vi "MasterSlaveDAQ-SplitSlave.vi"() -> ()   [LabVIEW 2014]
uses:
  subVIs/SlaveState.ctl
  subVIs/SlaveStateData.ctl
  <vilib>/Utility/error.llb/DialogType.ctl
  <vilib>/DAQmx/read.llb/DAQmx Read (Analog Wfm 1Chan NSamp).vi
  <resource>/objmgr/daqmx.rc
panel:
  out "Waveform Chart":waveform(dbl)(graph)
  in  "Acquire Data":bool
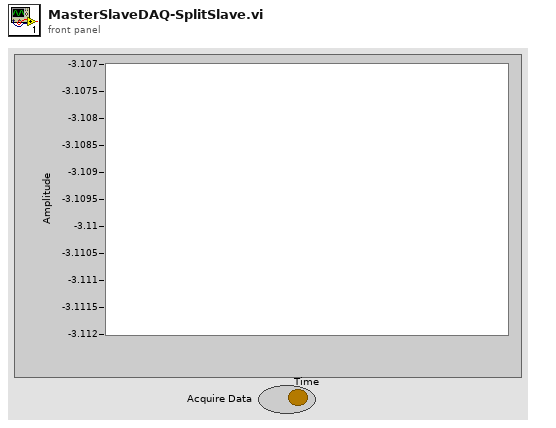
[diagram p1: front panel]
types:
  T1 = typedef "SlaveStateData.ctl" = cluster{"New State":T2, "DAQ Ref":refnum<k21>, "File Ref":refnum<file>}
  T2 = typedef "SlaveState.ctl" = enum16{"Init", "Idle", "CheckError", "Finalize", "StartDAQ", "AcquireAndLog", "StopDAQ", "UpdateFile"}
  T3 = typedef "DialogType.ctl" = u16
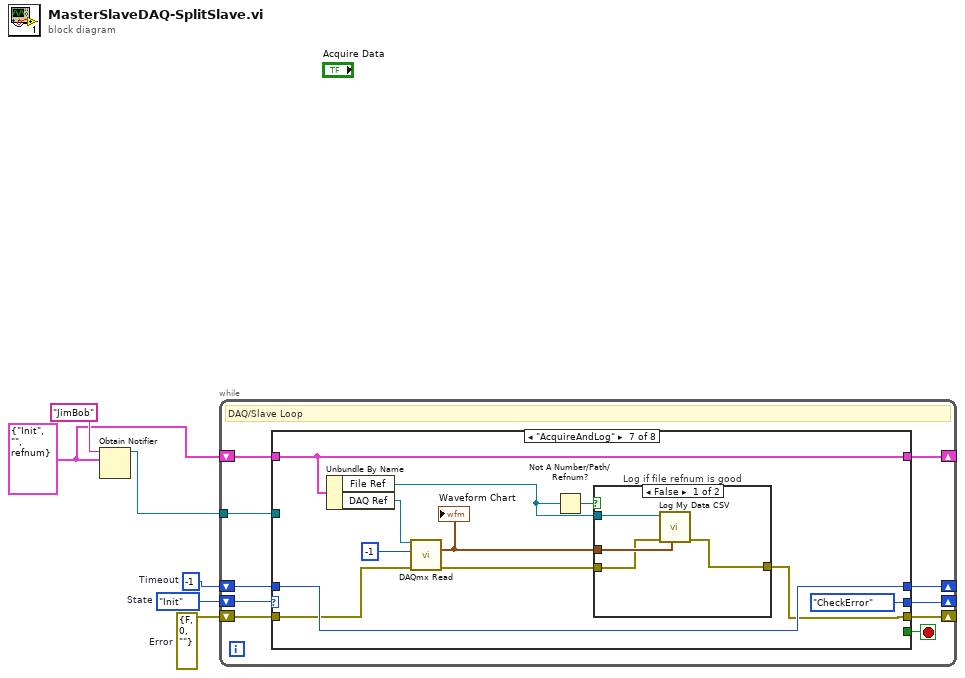
[diagram p0: block diagram]
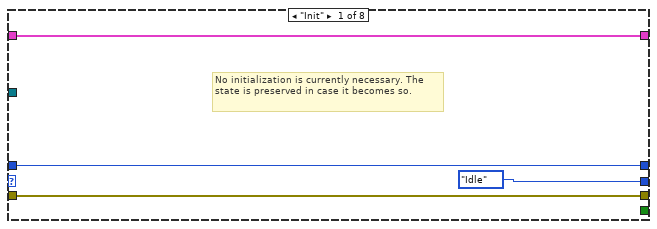
[diagram p2: hidden frame]
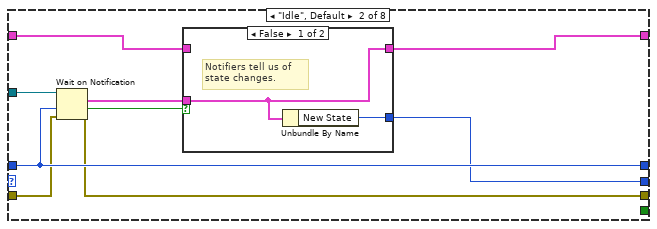
[diagram p3: hidden frame]
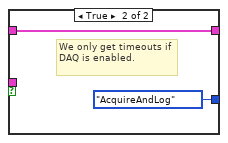
[diagram p4: hidden frame]
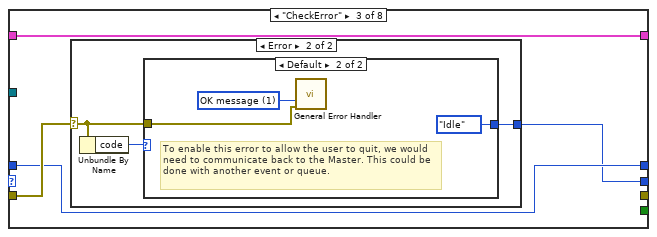
[diagram p5: hidden frame]
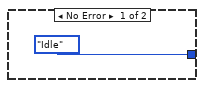
[diagram p6: hidden frame]
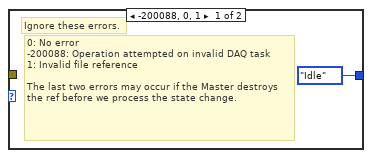
[diagram p7: hidden frame]
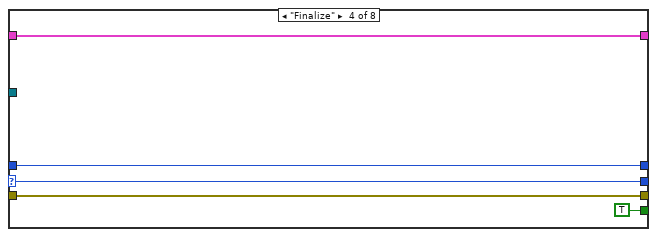
[diagram p8: hidden frame]
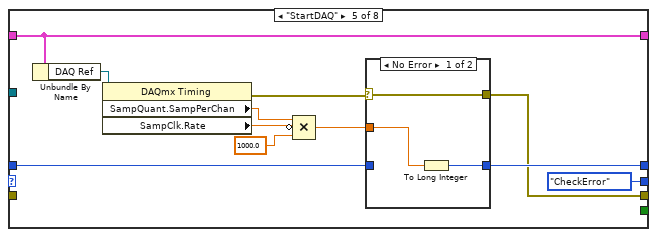
[diagram p9: hidden frame]
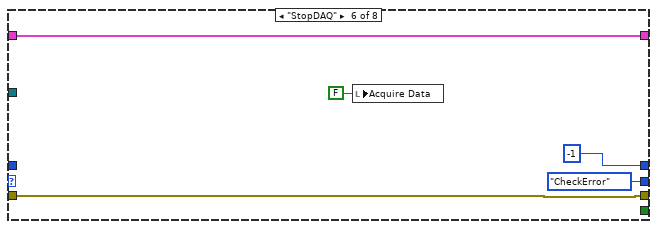
[diagram p11: hidden frame]
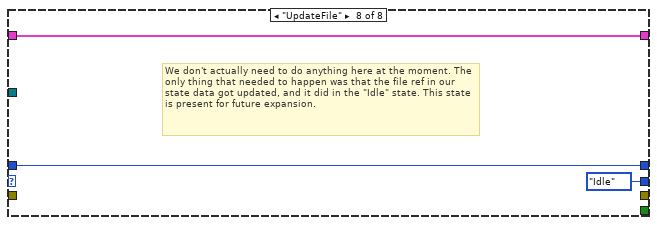
[diagram p13: hidden frame]
diagram:
  w1 = T1 {"New State"=enum."Init", "DAQ Ref"="", "File Ref"=refnum}
  w4 = errorcluster {"status"=FALSE, "code"=0, "source"=""}  # Error
  w5 = -1  # Timeout
  w6 = SlaveState."Init"  # State
  n1 = Obtain Notifier(name (unnamed)="JimBob", notification data type=w1) -> (notifier out=w2:refnum<notifier>)  [unwired: 2 in, 2 out]
  n2 = while {
    tunnel: w2 -> [w15]
    shift-right: [w14] -> _
    shift-left: w6 -> [w16]
    shift-right: [w10] -> _
    shift-left: w1 -> [w13]
    shift-right: [w11] -> _
    shift-left: w5 -> [w12]
    shift-right: [w8] -> _
    shift-left: w4 -> [w9]
    stop <- w7 stop-if-true
    # "DAQ/Slave Loop"
    n3 = case shown="\"AcquireAndLog\"" w16 {
      selector: w16 -> [_ _ _ w47 _ _ _ _]
      tunnel: w15 -> [_ w29 _ _ _ _ _ _]
      tunnel: [SlaveState."Idle" ("New State") w22 w34 w47 SlaveState."CheckError" ("State") SlaveState."CheckError" ("State") SlaveState."CheckError" ("State") SlaveState."Idle" ("State")] -> w14
      tunnel: w13 -> [w18 w24 w37 w49 w58 w71 w76 w90]
      tunnel: w12 -> [w19 w28 w35 w48 w60 _ w77 w89]
      tunnel: [w19 w28 w35 w48 w61 -1 w77 w89] -> w11
      tunnel: [w18 w21 w37 w49 w58 w71 w76 w90] -> w10
      tunnel: w9 -> [w17 w26 w36 w46 _ w67 w74 _]
      tunnel: [w17 w27 _ w46 w59 w67 w73 _] -> w8
      tunnel: [_ _ _ TRUE _ _ _ _] -> w7
      frame "Init" {
        # "No initialization is currently necessary. The state is preserved in case it becomes so."
      }
      frame "Idle", Default {
        n4 = Wait on Notification(notifier=w29, timeout in ms (-1)=w28, error in (no error)=w26) -> (notification=w23:T1, timed out?=w25:bool, error out=w27:errorcluster)  [unwired: 1 in, 1 out]
        n5 = case shown="False" w25 {
          tunnel: w24 -> [_ w33]
          tunnel: w23 -> [w30 _]
          tunnel: [w31 SlaveState."AcquireAndLog" ("New State")] -> w22
          tunnel: [w30 w33] -> w21
          frame False {
            # "Notifiers tell us of state changes."
            n6 = Unbundle By Name(w30) -> ("New State"=w31:T2)
          }
          frame True {
            # "We only get timeouts if DAQ is enabled."
          }
        }
      }
      frame "CheckError" {
        n7 = case shown="Error" w36 {
          selector: w36 -> [_ w40]
          tunnel: [SlaveState."Idle" ("State") w41] -> w34
          frame No Error {
          }
          frame Error {
            n8 = Unbundle By Name(w40) -> ("code"=w39:i32)
            n9 = case shown="Default" w39 {
              tunnel: [SlaveState."Idle" ("State") SlaveState."Idle" ("State")] -> w41
              tunnel: w40 -> [_ w44]
              frame -200088, 0, 1 {
                # "0: No error\n-200088: Operation attempted on invalid DAQ task\n1: Invalid file reference\n\nThe last two errors may occur if the Master destroys the ref before we process the state change."
                # "Ignore these errors."
              }
              frame Default {
                w45 = T3 1 items=["no dialog", "OK message", "continue or stop message", "OK message + warnings", "continue/stop + warnings"] ("type of dialog (OK msg:1)")
                # "To enable this error to allow the user to quit, we would need to communicate back to the Master. This could be done with another event or queue."
                n10 = call <vilib>:"General Error Handler.vi"("type of dialog (OK msg:1)"=w45, "error in (no error)"=w44) -> ()  [unwired: 9 in, 5 out]
              }
            }
          }
        }
      }
      frame "Finalize" {
      }
      frame "StartDAQ" {
        n11 = Unbundle By Name(w58) -> ("DAQ Ref"=w57:refnum<k21>)
        n12 = property class="DAQmx Timing"(reference=w57) -> (error out=w55:errorcluster, "SampQuant.SampPerChan"=w54:dbl, "SampClk.Rate"=w53:dbl)  [unwired: 1 in, 1 out]
        n13 = Compound Arithmetic op=MULTIPLY(w54, invert w53, 1000.0 ("value")) -> (w51:dbl)
        n14 = case shown="No Error" w55 {
          selector: w55 -> [w63 w66]
          tunnel: [w64 w65] -> w61
          tunnel: [w63 w66] -> w59
          tunnel: w60 -> [_ w65]
          tunnel: w51 -> [w62 _]
          frame No Error {
            n15 = To Long Integer(number=w62) -> (32bit integer=w64:i32)
          }
          frame Error {
          }
        }
      }
      frame "StopDAQ" {
        n16 = local write "Acquire Data"(FALSE ("Acquire Data")) -> ()
      }
      frame "AcquireAndLog" {
        n17 = Unbundle By Name(w76) -> ("File Ref"=w72:refnum<file>, "DAQ Ref"=w75:refnum<k21>)
        n18 = call-poly <vilib>:"DAQmx Read.vi"("task/channels in"=w75, "number of samples per channel"=-1, "error in"=w74) -> ("data"=w78:waveform(dbl), "error out"=w79:errorcluster)  [unwired: 10 in, 1 out]
        "Waveform Chart" <- w78
        n19 = Not A Number/Path/Refnum?(number/path/refnum=w72) -> (NaN/Path/Refnum?=w80:bool)
        n20 = case "Log if file refnum is good" shown="False" w80 {
          tunnel: w79 -> [w83 w87]
          tunnel: w72 -> [w86 _]
          tunnel: w78 -> [w85 _]
          tunnel: [w84 w87] -> w73
          frame False {
            n21 = call "Log My Data CSV.vi"("Data"=w85, "error in"=w83, "file refnum"=w86) -> ("error out"=w84:errorcluster)  [unwired: 7 in, 1 out]
          }
          frame True {
          }
        }
      }
      frame "UpdateFile" {
        # "We don't actually need to do anything here at the moment. The only thing that needed to happen was that the file ref in our state data got updated, and it did in the \"Idle\" state. This state is present for future expansion."
      }
    }
  }
